vi "ListFiles.vi"(11 "Folder":path) -> (3 "TDMS":string[](array[string]))   [LabVIEW 2019]
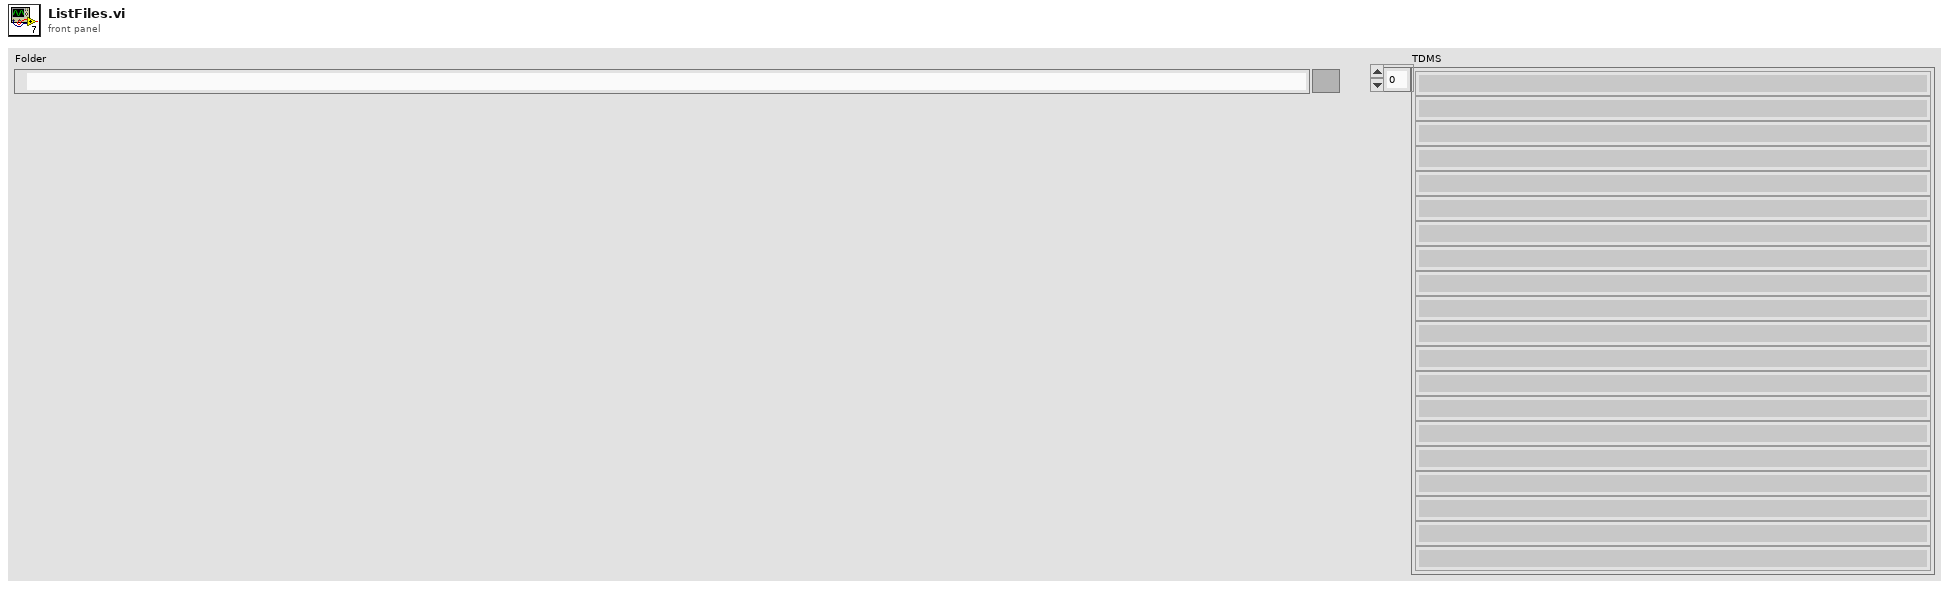
[diagram p1: front panel]
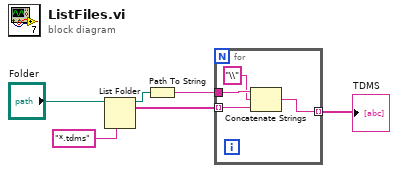
[diagram p0: block diagram]
diagram:
  n1 = List Folder(path="Folder", pattern="*.tdms") -> (path out=w4:path, filenames=w6:string[])  [unwired: 2 in, 2 out]
  n2 = Path To String(path=w4) -> (string=w5:string)
  n3 = for {
    tunnel: w6 -> [w8] mode=indexing
    tunnel: [w10] -> w3 mode=indexing
    tunnel: w5 -> [w9]
    n4 = Concatenate Strings(w9, "\\" ("string"), w8) -> (w10:string)
  }
  "TDMS" <- w3
